vi "ExecuteCommands.vi"(8 "error in (no error)":errorcluster, 11 "Control in":refnum<class "Control-Server.lvclass">) -> (0 "error out":errorcluster, 3 "Control out":refnum<class "Control-Server.lvclass">)   [LabVIEW 2015, in "Control-Server.lvclass"]
uses:
  Control-Server.lvclass
  dependecies/ControlsVIs/Clusters-def/Message types.ctl
  dependecies/ControlsVIs/Clusters-def/Standard Command.ctl
  dependecies/ControlsVIs/Clusters-def/ProtypeCommand-CommandUnknown.ctl
  dependecies/ControlsVIs/Clusters-def/SERVER-Commands.ctl
  dependecies/ControlsVIs/Clusters-def/DL-Reply-to-Connect.ctl
  Delay Line/DelayLine.lvclass
  Control-Server.lvclass/Control-Server.ctl
  dependecies/ControlsVIs/Clusters-def/Det-Reply-to-Connect.ctl
  Detector/Detector.lvclass
  dependecies/ControlsVIs/Clusters-def/DAQmx-Reply-to-Connect.ctl
  DAQmxTasks/DAQmxTaskContainer_General/DAQmxTaksContainer_General.lvclass
  dependecies/ControlsVIs/Clusters-def/OSc-Reply-to-Connect.ctl
  Oscilloscope/Oscilloscope.lvclass
  dependecies/ControlsVIs/Clusters-def/TEST-def.ctl
  <vilib>/regexp/Match Regular Expression.xnode
  GeneralFunctionality/GeneralFunctionality.lvclass
  DB/DB.lvclass
  Message/Message.lvclass
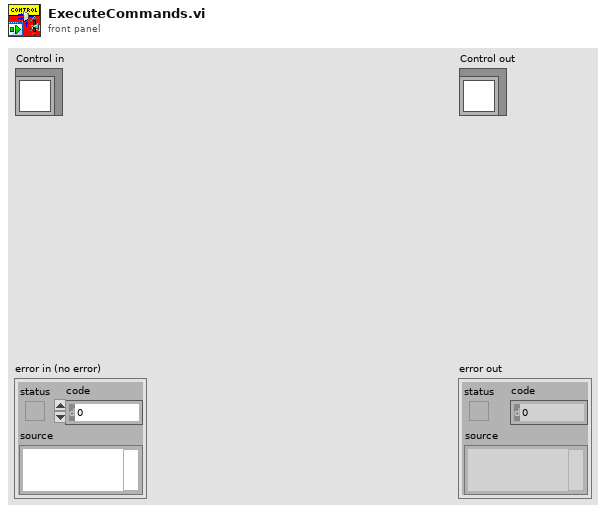
[diagram p1: front panel]
types:
  T1 = typedef "Message types.ctl" = string
  T2 = typedef "Standard Command.ctl" = cluster{"command":string, "data":variant}
  T3 = typedef "ProtypeCommand-CommandUnknown.ctl" = cluster{"error in (no error)":errorcluster}
  T4 = typedef "Control-Server.lvclass/SERVER-Commands.ctl" = string
  T5 = typedef "DelayLine.lvclass/DL-Reply-to-Connect.ctl" = cluster{"On/Off":bool, "error":errorcluster, "DelayLine.lvclass":refnum<class "DelayLine.lvclass">}
  T6 = typedef "Detector.lvclass/Det-Reply-to-Connect.ctl" = cluster{"On/Off":bool, "error":errorcluster, "Detector":refnum<class "Detector.lvclass">}
  T7 = typedef "DAQmxTaksContainer_General.lvclass/DAQmx-Reply-to-Connect.ctl" = cluster{"On/Off":bool, "error":errorcluster, "DAQmxTaskContainer_General":refnum<class "DAQmxTaksContainer_General.lvclass">}
  T8 = typedef "Oscilloscope.lvclass/OSc-Reply-to-Connect.ctl" = cluster{"On/Off":bool, "error":errorcluster, "Oscilloscope.lvclass":refnum<class "Oscilloscope.lvclass">}
  T9 = typedef "TEST-def.ctl" = cluster{"data":cluster{i32[], dbl[]}[]}
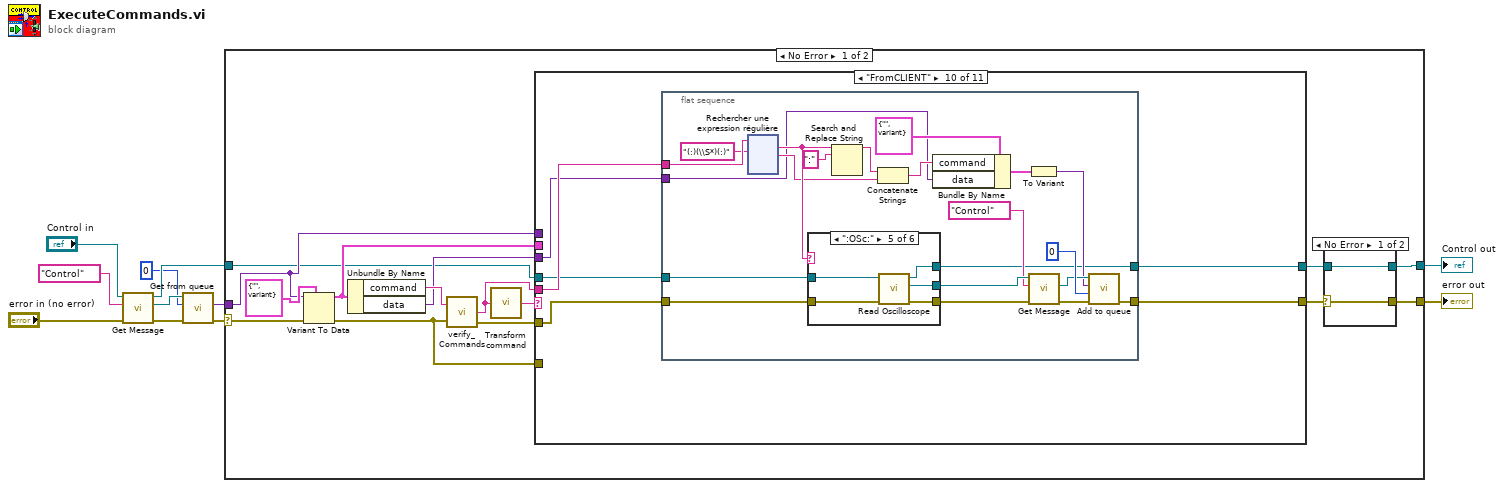
[diagram p0: block diagram]
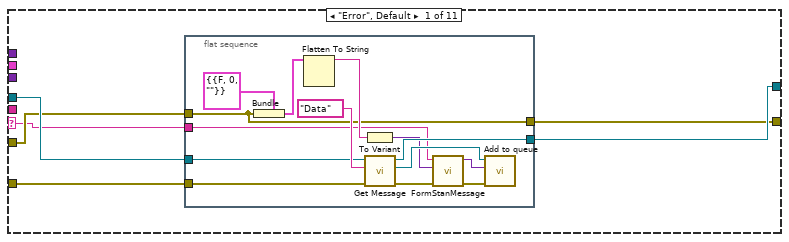
[diagram p2: hidden frame]
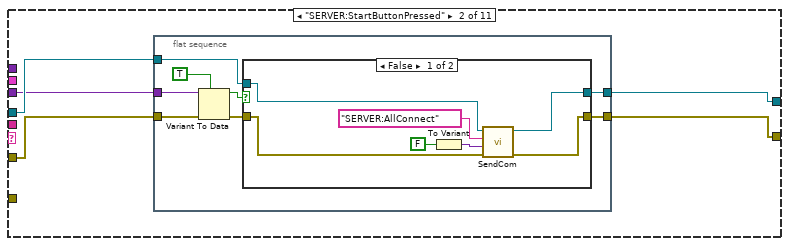
[diagram p3: hidden frame]
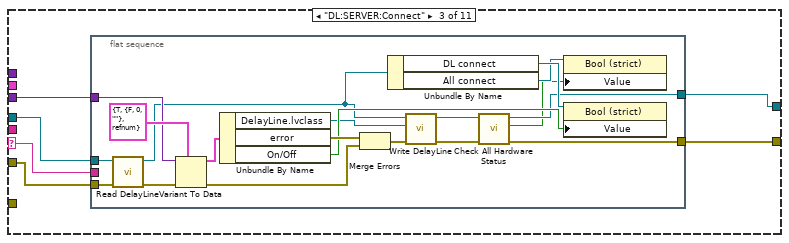
[diagram p5: hidden frame]
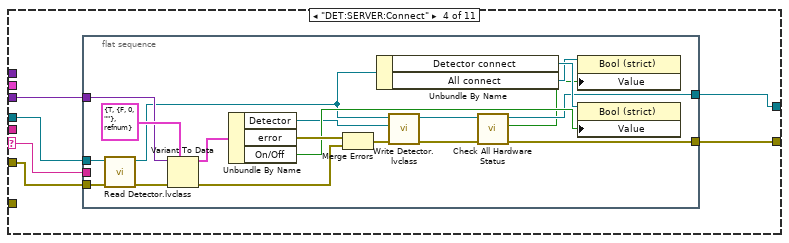
[diagram p6: hidden frame]
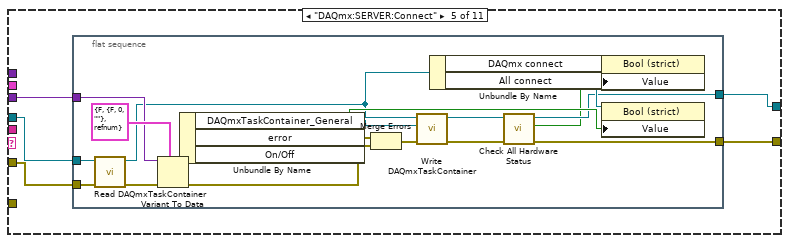
[diagram p7: hidden frame]
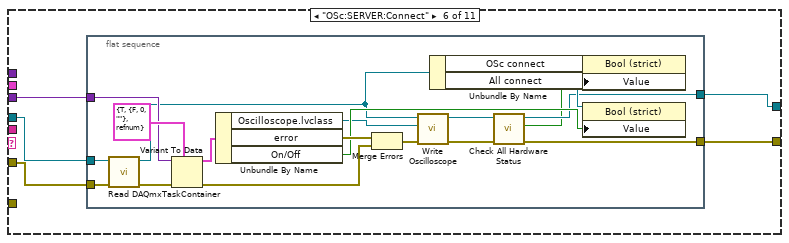
[diagram p8: hidden frame]
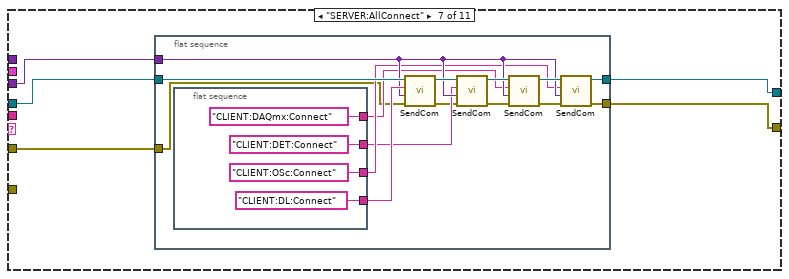
[diagram p9: hidden frame]
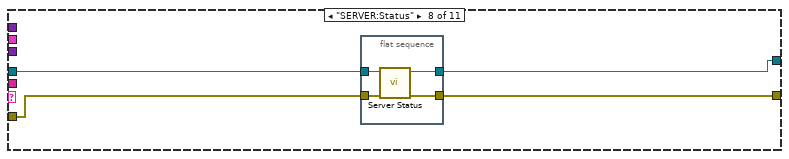
[diagram p10: hidden frame]
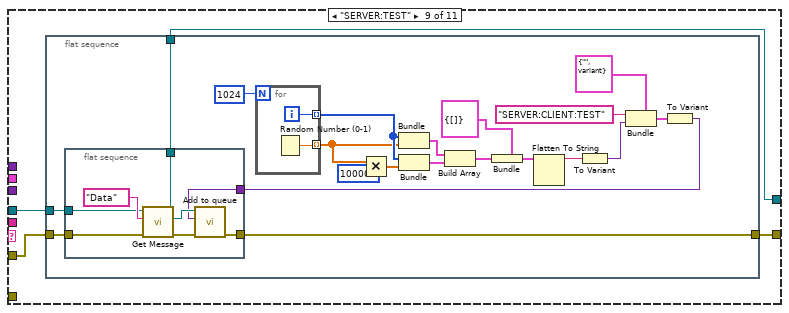
[diagram p11: hidden frame]
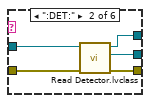
[diagram p13: hidden frame]
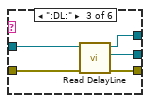
[diagram p14: hidden frame]
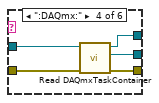
[diagram p15: hidden frame]
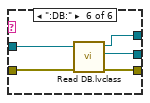
[diagram p16: hidden frame]
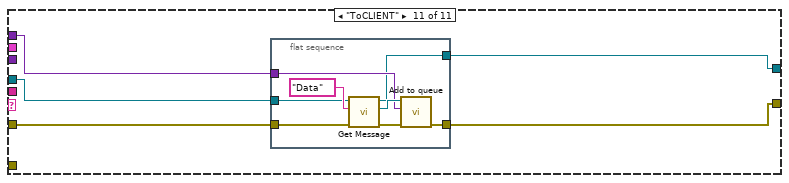
[diagram p17: hidden frame]
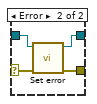
[diagram p18: hidden frame]
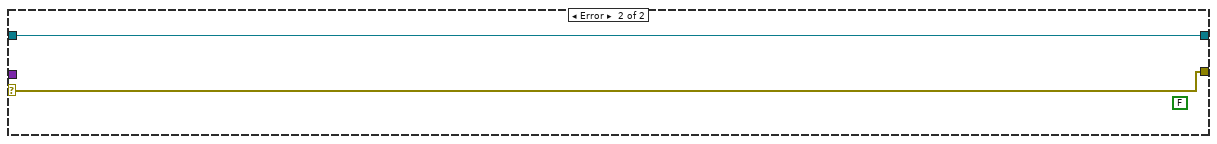
[diagram p19: hidden frame]
diagram:
  n1 = call "Get Message.vi"("error in (no error)"="error in (no error)", "Message type"=T1 "Control", "GeneralFunctionality en entrée"="Control in") -> ("error out"=w7:errorcluster, "Message.lvclass"=w4:refnum<class "Message.lvclass">, "GeneralFunctionality en sortie"=w6:refnum<class "Control-Server.lvclass">)  [unwired: 6 in]
  n2 = call "Get from queue.vi"("error in (no error)"=w7, "timeout in ms (-1)"=0, "Message in"=w4) -> ("error out"=w1:errorcluster, "Data"=w5:variant)  [unwired: 5 in, 2 out]
  n3 = case shown="No Error" w1 {
    selector: w1 -> [w13 w420]
    tunnel: w6 -> [w12 w421]
    tunnel: [w24 w421] -> w9
    tunnel: [w23 w420] -> w8
    tunnel: w5 -> [w14 _]
    frame No Error {
      n4 = Variant To Data(error in=w13, type=T2 {"command"="", "data"=variant} ("input cluster"), Variant=w14) -> (data=w21:T2, error out=w18:errorcluster)
      n5 = Unbundle By Name(w21) -> ("command"=w19:string, "data"=w16:variant)
      n6 = call "verify_Commands.vi"("Command"=w19, "error in"=w18) -> ("Command out"=w15:string, "error out"=w20:errorcluster)  [unwired: 1 out]
      n7 = call "Transform command.vi"("Command in"=w15) -> ("Comamnd out"=w17:string)
      n8 = case shown="\"FromCLIENT\"" w17 {
        selector: w17 -> [w29 _ w70 w95 _ _ _ _ _ _ _]
        tunnel: w20 -> [w31 w50 w73 w98 w123 w147 w167 w194 w200 w235 w404]
        tunnel: w12 -> [w32 w51 w74 w99 w122 w146 w171 w191 w201 w236 w405]
        tunnel: [w30 w49 w71 w96 w120 w144 w170 w192 w199 w233 w401] -> w25
        tunnel: [w28 w48 w72 w97 w121 w145 w169 w193 w202 w238 w403] -> w22
        tunnel: w21 -> [_ _ _ _ _ _ _ _ _ _ _]
        tunnel: w18 -> [w27 _ _ _ _ _ _ _ _ _ _]
        tunnel: w16 -> [_ w47 w69 w94 w119 w143 w168 _ _ w234 _]
        tunnel: w15 -> [_ _ _ _ _ _ _ _ _ w237 _]
        tunnel: w14 -> [_ _ _ _ _ _ _ _ _ _ w402]
        frame "Error", Default {
          n9 = flat-sequence {
            tunnel: w32 -> [w41]
            tunnel: w31 -> [w34]
            tunnel: [w40] -> w30
            tunnel: w29 -> [w39]
            tunnel: [w34] -> w28
            tunnel: w27 -> [w33]
            frame #0 {
              n10 = Bundle(cluster=T3 {"error in (no error)"={"status"=FALSE, "code"=0, "source"=""}}, "error in (no error)"=w34) -> (w46:T3)
              n11 = Flatten To String(anything=w46) -> (data string=w45:string)  [unwired: 3 in, 2 out]
              n12 = To Variant(anything=w45) -> (Variant=w38:variant)
              n13 = call "Get Message.vi"("error in (no error)"=w33, "Message type"=T1 "Data", "GeneralFunctionality en entrée"=w41) -> ("error out"=w37:errorcluster, "Message.lvclass"=w43:refnum<class "Message.lvclass">, "GeneralFunctionality en sortie"=w40:refnum<class "Control-Server.lvclass">)  [unwired: 6 in]
              n14 = call "FormStanMessage.vi"("error in"=w37, "data"=w38, "Command"=w39) -> ("error out"=w36:errorcluster, "message"=w35:variant)  [unwired: 7 in]
              n15 = call "Add to queue.vi"("error in (no error)"=w36, "Data"=w35, "Message in"=w43) -> ()  [unwired: 7 in, 2 out]
            }
          }
        }
        frame "SERVER:StartButtonPressed" {
          n16 = flat-sequence {
            tunnel: w51 -> [w57]
            tunnel: w50 -> [w56]
            tunnel: [w54] -> w49
            tunnel: [w53] -> w48
            tunnel: w47 -> [w52]
            frame #0 {
              n17 = Variant To Data(error in=w56, type=TRUE, Variant=w52) -> (data=w58:bool, error out=w55:errorcluster)
              n18 = case shown="False" w58 {
                tunnel: w57 -> [w64 w68]
                tunnel: w55 -> [w63 w67]
                tunnel: [w61 w68] -> w54
                tunnel: [w60 w67] -> w53
                frame False {
                  n19 = To Variant(anything=FALSE) -> (Variant=w65:variant)
                  n20 = call "SendCom.vi"("error in (no error)"=w63, "data"=w65, "Command"=T4 "SERVER:AllConnect" ("Commands"), "Control in"=w64) -> ("error out"=w60:errorcluster, "Control out"=w61:refnum<class "Control-Server.lvclass">)  [unwired: 6 in]
                }
                frame True {
                }
              }
            }
          }
        }
        frame "DL:SERVER:Connect" {
          n21 = flat-sequence {
            tunnel: w74 -> [w84]
            tunnel: w73 -> [w83]
            tunnel: [w81] -> w72
            tunnel: [w80] -> w71
            tunnel: w70 -> [_]
            tunnel: w69 -> [w79]
            frame #0 {
              n22 = call "Read DelayLine.vi"("error in (no error)"=w83, "Control in"=w84) -> ("error out"=w85:errorcluster, "Control out"=w75:refnum<class "Control-Server.lvclass">)  [unwired: 7 in, 1 out]
              n23 = Variant To Data(error in=w85, type=T5 {"On/Off"=TRUE, "error"={"status"=FALSE, "code"=0, "source"=""}, "DelayLine.lvclass"=refnum}, Variant=w79) -> (data=w87:T5, error out=w91:errorcluster)
              n24 = Unbundle By Name(w87) -> ("DelayLine.lvclass"=w88:refnum<class "DelayLine.lvclass">, "error"=w90:errorcluster, "On/Off"=w89:bool)
              n25 = Merge Errors(w90, w91) -> (w92:errorcluster)
              n26 = Unbundle By Name(w75) -> ("DL connect"=w93:refnum<vi>, "All connect"=w77:refnum<vi>)
              n27 = call "Write DelayLine.vi"("error in (no error)"=w92, "DelayLine.lvclass"=w88, "Control in"=w75) -> ("error out"=w78:errorcluster, "Control out"=w82:refnum<class "Control-Server.lvclass">)  [unwired: 7 in]
              n28 = call "Check All Hardware Status.vi"("error in (no error)"=w78, "Control en entrée"=w82) -> ("error out"=w81:errorcluster, "HARDWARE"=w76:bool, "Control en sortie"=w80:refnum<class "Control-Server.lvclass">)  [unwired: 7 in]
              n29 = property class="Bool (strict)"(reference=w77, "Value"=w76) -> ()  [unwired: 1 in, 2 out]
              n30 = property class="Bool (strict)"(reference=w93, "Value"=w89) -> ()  [unwired: 1 in, 2 out]
            }
          }
        }
        frame "DET:SERVER:Connect" {
          n31 = flat-sequence {
            tunnel: w98 -> [w110]
            tunnel: w99 -> [w112]
            tunnel: [w106] -> w97
            tunnel: [w105] -> w96
            tunnel: w95 -> [_]
            tunnel: w94 -> [w103]
            frame #0 {
              n32 = call "Read Detector.lvclass.vi"("error in (no error)"=w110, "Control in"=w112) -> ("error out"=w111:errorcluster, "Control out"=w100:refnum<class "Control-Server.lvclass">)  [unwired: 7 in, 1 out]
              n33 = Variant To Data(error in=w111, type=T6 {"On/Off"=TRUE, "error"={"status"=FALSE, "code"=0, "source"=""}, "Detector"=refnum}, Variant=w103) -> (data=w114:T6, error out=w117:errorcluster)
              n34 = Unbundle By Name(w114) -> ("Detector"=w108:refnum<class "Detector.lvclass">, "error"=w116:errorcluster, "On/Off"=w115:bool)
              n35 = Merge Errors(w116, w117) -> (w109:errorcluster)
              n36 = Unbundle By Name(w100) -> ("Detector connect"=w118:refnum<vi>, "All connect"=w102:refnum<vi>)
              n37 = call "Write Detector.lvclass.vi"("error in (no error)"=w109, "Detector.lvclass"=w108, "Control in"=w100) -> ("error out"=w104:errorcluster, "Control out"=w107:refnum<class "Control-Server.lvclass">)  [unwired: 7 in]
              n38 = call "Check All Hardware Status.vi"("error in (no error)"=w104, "Control en entrée"=w107) -> ("error out"=w106:errorcluster, "HARDWARE"=w101:bool, "Control en sortie"=w105:refnum<class "Control-Server.lvclass">)  [unwired: 7 in]
              n39 = property class="Bool (strict)"(reference=w102, "Value"=w101) -> ()  [unwired: 1 in, 2 out]
              n40 = property class="Bool (strict)"(reference=w118, "Value"=w115) -> ()  [unwired: 1 in, 2 out]
            }
          }
        }
        frame "DAQmx:SERVER:Connect" {
          n41 = flat-sequence {
            tunnel: w123 -> [w133]
            tunnel: w122 -> [w132]
            tunnel: [w130] -> w121
            tunnel: [w129] -> w120
            tunnel: w119 -> [w127]
            frame #0 {
              n42 = call-dynamic "Read DAQmxTaskContainer.vi"("error in (no error)"=w133, "Control in"=w132) -> ("error out"=w136:errorcluster, "Control out"=w124:refnum<class "Control-Server.lvclass">)  [unwired: 7 in, 1 out]
              n43 = Variant To Data(error in=w136, type=T7 {"On/Off"=FALSE, "error"={"status"=FALSE, "code"=0, "source"=""}, "DAQmxTaskContainer_General"=refnum}, Variant=w127) -> (data=w138:T7, error out=w141:errorcluster)
              n44 = Unbundle By Name(w138) -> ("DAQmxTaskContainer_General"=w135:refnum<class "DAQmxTaksContainer_General.lvclass">, "error"=w140:errorcluster, "On/Off"=w139:bool)
              n45 = Merge Errors(w140, w141) -> (w134:errorcluster)
              n46 = call-dynamic "Write DAQmxTaskContainer.vi"("error in (no error)"=w134, "DAQmxTaksContainer_General.lvclass"=w135, "Control in"=w124) -> ("error out"=w128:errorcluster, "Control out"=w131:refnum<class "Control-Server.lvclass">)  [unwired: 7 in]
              n47 = Unbundle By Name(w124) -> ("DAQmx connect"=w142:refnum<vi>, "All connect"=w126:refnum<vi>)
              n48 = call "Check All Hardware Status.vi"("error in (no error)"=w128, "Control en entrée"=w131) -> ("error out"=w130:errorcluster, "HARDWARE"=w125:bool, "Control en sortie"=w129:refnum<class "Control-Server.lvclass">)  [unwired: 7 in]
              n49 = property class="Bool (strict)"(reference=w126, "Value"=w125) -> ()  [unwired: 1 in, 2 out]
              n50 = property class="Bool (strict)"(reference=w142, "Value"=w139) -> ()  [unwired: 1 in, 2 out]
            }
          }
        }
        frame "OSc:SERVER:Connect" {
          n51 = flat-sequence {
            tunnel: w147 -> [w157]
            tunnel: w146 -> [w156]
            tunnel: [w154] -> w145
            tunnel: [w153] -> w144
            tunnel: w143 -> [w151]
            frame #0 {
              n52 = call-dynamic "Read DAQmxTaskContainer.vi"("error in (no error)"=w157, "Control in"=w156) -> ("error out"=w160:errorcluster, "Control out"=w148:refnum<class "Control-Server.lvclass">)  [unwired: 7 in, 1 out]
              n53 = Variant To Data(error in=w160, type=T8 {"On/Off"=TRUE, "error"={"status"=FALSE, "code"=0, "source"=""}, "Oscilloscope.lvclass"=refnum}, Variant=w151) -> (data=w162:T8, error out=w165:errorcluster)
              n54 = Unbundle By Name(w162) -> ("Oscilloscope.lvclass"=w159:refnum<class "Oscilloscope.lvclass">, "error"=w164:errorcluster, "On/Off"=w163:bool)
              n55 = Merge Errors(w164, w165) -> (w158:errorcluster)
              n56 = call "Write Oscilloscope.vi"("error in (no error)"=w158, "Oscilloscope.lvclass"=w159, "Control-Server en entrée"=w148) -> ("error out"=w152:errorcluster, "Control-Server en sortie"=w155:refnum<class "Control-Server.lvclass">)  [unwired: 7 in]
              n57 = Unbundle By Name(w148) -> ("OSc connect"=w166:refnum<vi>, "All connect"=w150:refnum<vi>)
              n58 = call "Check All Hardware Status.vi"("error in (no error)"=w152, "Control en entrée"=w155) -> ("error out"=w154:errorcluster, "HARDWARE"=w149:bool, "Control en sortie"=w153:refnum<class "Control-Server.lvclass">)  [unwired: 7 in]
              n59 = property class="Bool (strict)"(reference=w150, "Value"=w149) -> ()  [unwired: 1 in, 2 out]
              n60 = property class="Bool (strict)"(reference=w166, "Value"=w163) -> ()  [unwired: 1 in, 2 out]
            }
          }
        }
        frame "SERVER:AllConnect" {
          n61 = flat-sequence {
            tunnel: w171 -> [w184]
            tunnel: [w181] -> w170
            tunnel: [w180] -> w169
            tunnel: w168 -> [w177]
            tunnel: w167 -> [w173]
            frame #0 {
              n62 = flat-sequence {
                tunnel: ["CLIENT:DL:Connect" ("Command")] -> w186
                tunnel: ["CLIENT:OSc:Connect" ("Command")] -> w176
                tunnel: ["CLIENT:DET:Connect" ("Command")] -> w175
                tunnel: ["CLIENT:DAQmx:Connect" ("Command")] -> w174
                frame #0 {
                }
              }
              n63 = call "SendCom.vi"("error in (no error)"=w173, "data"=w177, "Command"=w186, "Control in"=w184) -> ("error out"=w172:errorcluster, "Control out"=w185:refnum<class "Control-Server.lvclass">)  [unwired: 6 in]
              n64 = call "SendCom.vi"("error in (no error)"=w172, "data"=w177, "Command"=w175, "Control in"=w185) -> ("error out"=w178:errorcluster, "Control out"=w183:refnum<class "Control-Server.lvclass">)  [unwired: 6 in]
              n65 = call "SendCom.vi"("error in (no error)"=w178, "data"=w177, "Command"=w174, "Control in"=w183) -> ("error out"=w179:errorcluster, "Control out"=w182:refnum<class "Control-Server.lvclass">)  [unwired: 6 in]
              n66 = call "SendCom.vi"("error in (no error)"=w179, "data"=w177, "Command"=w176, "Control in"=w182) -> ("error out"=w180:errorcluster, "Control out"=w181:refnum<class "Control-Server.lvclass">)  [unwired: 6 in]
            }
          }
        }
        frame "SERVER:Status" {
          n67 = flat-sequence {
            tunnel: w194 -> [w195]
            tunnel: [w198] -> w193
            tunnel: [w197] -> w192
            tunnel: w191 -> [w196]
            frame #0 {
              n68 = call "Server Status.vi"("entrée d'erreur (pas d'erreur)"=w195, "Control en entrée"=w196) -> ("sortie d'erreur"=w198:errorcluster, "Control en sortie"=w197:refnum<class "Control-Server.lvclass">)  [unwired: 8 in]
            }
          }
        }
        frame "SERVER:TEST" {
          n69 = flat-sequence {
            tunnel: [w222] -> w202
            tunnel: w201 -> [w221]
            tunnel: w200 -> [w220]
            tunnel: [w203] -> w199
            frame #0 {
              n70 = flat-sequence {
                tunnel: [w232] -> w222
                tunnel: w221 -> [w228]
                tunnel: w220 -> [w227]
                tunnel: w209 -> [w226]
                tunnel: [w225] -> w203
                frame #0 {
                  n71 = call "Get Message.vi"("error in (no error)"=w227, "Message type"=T1 "Data", "GeneralFunctionality en entrée"=w228) -> ("error out"=w230:errorcluster, "Message.lvclass"=w229:refnum<class "Message.lvclass">, "GeneralFunctionality en sortie"=w225:refnum<class "Control-Server.lvclass">)  [unwired: 6 in]
                  n72 = call "Add to queue.vi"("error in (no error)"=w230, "Data"=w226, "Message in"=w229) -> ("error out"=w232:errorcluster)  [unwired: 7 in, 1 out]
                }
              }
              n73 = for {
                N: 1024 -> [_]
                tunnel: [w224] -> w218 mode=indexing
                tunnel: [w223] -> w217 mode=indexing
                i -> [w224]
                n74 = Random Number (0-1)() -> (number: 0 to 1=w223:dbl)
              }
              n75 = Multiply(x=w217, y=100000 ("number: 0 to 1")) -> (x*y=w215:dbl[])
              n76 = Bundle(w218, w217) -> (w219:cluster{i32[], dbl[]})  [unwired: 1 in]
              n77 = Bundle(w218, w215) -> (w214:cluster{i32[], dbl[]})  [unwired: 1 in]
              n78 = Build Array(w219, w214) -> (w206:cluster{i32[], dbl[]}[])
              n79 = Bundle(cluster=T9 {"data"=[]} ("output cluster"), "data"=w206) -> (w204:T9)
              n80 = Flatten To String(anything=w204) -> (data string=w212:string)  [unwired: 3 in, 2 out]
              n81 = To Variant(anything=w212) -> (Variant=w211:variant)
              n82 = Bundle(cluster=T2 {"command"="", "data"=variant} ("input cluster"), "command"="SERVER:CLIENT:TEST", "data"=w211) -> (w210:T2)
              n83 = To Variant(anything=w210) -> (Variant=w209:variant)
            }
          }
        }
        frame "FromCLIENT" {
          n84 = flat-sequence {
            tunnel: [w259] -> w238
            tunnel: w237 -> [w258]
            tunnel: w236 -> [w256]
            tunnel: w235 -> [w255]
            tunnel: w234 -> [w242]
            tunnel: [w239] -> w233
            frame #0 {
              n85 = xnode "Rechercher une expression régulière"("input string"=w258, "regular expression"="(:)(\\S*)(:)") -> ("whole match"=w248:string, "after match"=w245:string)  [unwired: 4 in, 3 out]
              n86 = case shown="\":OSc:\"" w248 {
                tunnel: w256 -> [w260 w266 w270 w273 w281 w286]
                tunnel: w255 -> [w261 w263 w269 w276 w280 w283]
                tunnel: [w261 w264 w268 w275 w279 w284] -> w254
                tunnel: [_ w265 w271 w274 w278 w285] -> w253
                tunnel: [w260 w262 w267 w272 w277 w282] -> w239
                frame "False", Default {
                }
                frame ":DET:" {
                  n87 = call "Read Detector.lvclass.vi"("error in (no error)"=w263, "Control in"=w266) -> ("error out"=w264:errorcluster, "Detector.lvclass"=w265:refnum<class "Detector.lvclass">, "Control out"=w262:refnum<class "Control-Server.lvclass">)  [unwired: 7 in]
                }
                frame ":DL:" {
                  n88 = call "Read DelayLine.vi"("error in (no error)"=w269, "Control in"=w270) -> ("error out"=w268:errorcluster, "DelayLine.lvclass"=w271:refnum<class "DelayLine.lvclass">, "Control out"=w267:refnum<class "Control-Server.lvclass">)  [unwired: 7 in]
                }
                frame ":DAQmx:" {
                  n89 = call-dynamic "Read DAQmxTaskContainer.vi"("error in (no error)"=w276, "Control in"=w273) -> ("error out"=w275:errorcluster, "DAQmxTaksContainer_General.lvclass"=w274:refnum<class "DAQmxTaksContainer_General.lvclass">, "Control out"=w272:refnum<class "Control-Server.lvclass">)  [unwired: 7 in]
                }
                frame ":OSc:" {
                  n90 = call "Read Oscilloscope.vi"("error in (no error)"=w280, "Control-Server en entrée"=w281) -> ("error out"=w279:errorcluster, "Oscilloscope.lvclass"=w278:refnum<class "Oscilloscope.lvclass">, "Control-Server en sortie"=w277:refnum<class "Control-Server.lvclass">)  [unwired: 7 in]
                }
                frame ":DB:" {
                  n91 = call "Read DB.lvclass.vi"("error in (no error)"=w283, "Control-Server in"=w286) -> ("error out"=w284:errorcluster, "DB.lvclass"=w285:refnum<class "DB.lvclass">, "Control-Server out"=w282:refnum<class "Control-Server.lvclass">)  [unwired: 7 in]
                }
              }
              n92 = Search and Replace String(input string=w248, search string=":") -> (result string=w246:string)  [unwired: 6 in, 3 out]
              n93 = Concatenate Strings(w246, w245) -> (w243:string)
              n94 = Bundle By Name(cluster=T2 {"command"="", "data"=variant} ("input cluster"), "command"=w243, "data"=w242) -> (w241:T2)
              n95 = To Variant(anything=w241) -> (Variant=w240:variant)
              n96 = call "Get Message.vi"("error in (no error)"=w254, "Message type"=T1 "Control", "GeneralFunctionality en entrée"=w253) -> ("error out"=w249:errorcluster, "Message.lvclass"=w250:refnum<class "Message.lvclass">)  [unwired: 6 in, 1 out]
              n97 = call "Add to queue.vi"("error in (no error)"=w249, "timeout in ms (-1)"=0, "Data"=w240, "Message in"=w250) -> ("error out"=w259:errorcluster)  [unwired: 6 in, 1 out]
            }
          }
        }
        frame "ToCLIENT" {
          n98 = flat-sequence {
            tunnel: [w413] -> w403
            tunnel: w405 -> [w409]
            tunnel: w404 -> [w408]
            tunnel: w402 -> [w407]
            tunnel: [w406] -> w401
            frame #0 {
              n99 = call "Get Message.vi"("error in (no error)"=w408, "Message type"=T1 "Data", "GeneralFunctionality en entrée"=w409) -> ("error out"=w411:errorcluster, "Message.lvclass"=w410:refnum<class "Message.lvclass">, "GeneralFunctionality en sortie"=w406:refnum<class "Control-Server.lvclass">)  [unwired: 6 in]
              n100 = call "Add to queue.vi"("error in (no error)"=w411, "Data"=w407, "Message in"=w410) -> ("error out"=w413:errorcluster)  [unwired: 7 in, 1 out]
            }
          }
        }
      }
      n101 = case shown="No Error" w22 {
        selector: w22 -> [w414 w416]
        tunnel: w25 -> [w415 w419]
        tunnel: [w415 w418] -> w24
        tunnel: [w414 w417] -> w23
        frame No Error {
        }
        frame Error {
          n102 = call "Set error.vi"("error in (no error)"=w416, "Control-Server in"=w419) -> ("error out"=w417:errorcluster, "Control-Server out"=w418:refnum<class "Control-Server.lvclass">)  [unwired: 8 in]
        }
      }
    }
    frame Error {
      (unwired) FALSE
    }
  }
  "error out" <- w8
  "Control out" <- w9
